vi "Sequence.vi"(8 "error in (no error)":errorcluster, 11 "Message Queues in":T62) -> (0 "error out":errorcluster)   [LabVIEW 2018, in "Sequencing Library.lvlib"]
uses:
  Sequencing Library.lvlib
  Main/Main Queue Cluster.ctl
  support/Message Queue/Message Cluster.ctl
  Drag and Drop/State Cluster.ctl
  Drag and Drop/Thumbnail Cluster.ctl
  Drag and Drop/Object Cluster.ctl
  <vilib>/Utility/miscctls.llb/LVRectTypeDef.ctl
  Drag and Drop/Object Type Enum.ctl
  <vilib>/Utility/miscctls.llb/LVPositionTypeDef.ctl
  Config Module/Controls/Main Config Cluster.ctl
  OPC/OPC Module Config.ctl
  Scale Module Folder/Measure Instrument/State Enum.ctl
  <vilib>/Utility/miscctls.llb/LVPoint32TypeDef.ctl
  OPC/OPC Settings.ctl
  OPC/Variable Data Cluster.ctl
  <vilib>/OPCUA/controls/NodeId.ctl
  <vilib>/OPCUA/controls/OPC UA StatusCode.ctl
  <vilib>/OPCUA/controls/Subscription ID.ctl
  <vilib>/OPCUA/controls/OPC UA Client Refnum.ctl
  <vilib>/OPCUA/controls/Subscription Data Change.ctl
  <vilib>/OPCUA/controls/Data Type.ctl
  Feed Module/Controls/Feed Module Config Cluster.ctl
  Feed Module/Controls/Feed Module Settings Cluster.ctl
  Ismatec ISM 831C/Controls/Ismatech Settings Cluster.ctl
  Masterflex 7550-30/Controls/Settings Cluster.ctl
  Mettler Toledo/Controls/Settings Cluster.ctl
  Bronkhorst M13 Flow Meter/Settings Cluster.ctl
  Measure Instrument/PID 2 Parameters Cluster.ctl
  Measure Instrument/PID Input Enum.ctl
  Measure Instrument/PID 2 Output Enum.ctl
  Tacmina QI/Tacmina QI DAQ Setting.ctl
  KNF Pump/Settings Cluster plus SIMDOS.ctl
  ASIA Pump/Pump Settings.ctl
  VICI M50 Party Mode/Settings Cluster.ctl
  FLOM Pump/Settings Cluster.ctl
  SSI PR Class/SSI PR Settings Cluster.ctl
  TT Module/Controls/TT Module Config Cluster.ctl
  Acquisition/Hardware Configuration.ctl
  Acquisition/Task Cluster.ctl
  PT Module/Controls/PT Module Config Cluster.ctl
  Scale Module Folder/Feed Module/Controls/Scale Module Config Cluster.ctl
  Scale Module Folder/Feed Module/Controls/Scale Module Settings Cluster.ctl
  Pump Module Folder/Pump Module Config Cluster.ctl
  Pump Module Folder/Pump Module Settings Cluster.ctl
  LabJack Module/Controls/U3 Module Config Cluster.ctl
  Decoration Module/Decoration Module Config Cluster.ctl
  Flow Module Folder/Feed Module/Controls/Flow Module Config Cluster.ctl
  Flow Module Folder/Feed Module/Controls/Flow Module Settings Cluster.ctl
  TCU Module/TCU Module Folder/TCU Module Config Cluster.ctl
  TCU Module/TCU Module Folder/TCU Module Settings Cluster.ctl
  TCU Module/TCU Module Folder/Measure Instrument/Output Devices.ctl
  Huber TCU/Huber Settings.ctl
  Lauda Integral XT-150 TCU/Lauda Settings.ctl
  Julabo Type 1 TCU/Julabo Type 1 TCU Folder/Julabo FP-50 Settings.ctl
  Huber Unistat 410 TCU/Huber Unistat 410 Settings.ctl
  D-O Module Folder/Not Sure Where this is Used.ctl
  Squence Control.ctl
  D-O Module Folder/D-O Module Config Cluster.ctl
  D-O Module Folder/Valve Clusters.ctl
  D-O Module Folder/D-O Module Settings Cluster.ctl
  D-O Module Folder/D-O Device Settings Cluster.ctl
  VICI Electronic Actuator/VICI Electronic Actuator Settings.ctl
  Pressure Regulator Control Module/Pressure Regulator/Controls/4-20mA Module Config Cluster.ctl
  Pressure Regulator Control Module/Pressure Regulator/Controls/4-20mA Module Settings Cluster.ctl
  Pressure Transmitter/Pressure Transmitter Device Settings.ctl
  Pressure Reg Module/Pressure Regulator Device Settings.ctl
  Squence Update Cluster.ctl
  support/Message Queue/Enqueue Message (Single).vi
  support/Message Queue/Message Queue.lvlib
  support/Command Log VIs/Command Logging.lvlib
  Drag and Drop/Drag and Drop.lvlib
  Config Module/Config Module.lvlib
  TT Module/TT Module.lvlib
  Feed Module/Feed Module.lvlib
  Ismatec ISM 831C/Ismatec ISM 831C.lvlib
  Masterflex 7550-30/Masterflex 7550-30.lvlib
  Mettler Toledo/Mettler Toledo.lvlib
  Bronkhorst M13 Flow Meter/Bronkhorst M13 Flow Meter.lvlib
  Tacmina QI/Tacmina QI.lvlib
  KNF Pump/KNF SIMDOS.lvlib
  ASIA Pump.lvlib
  DAQ/DAQ.lvlib
  PT Module/PT Module.lvlib
  Scale Module Folder/Scale Module.lvlib
  Pump Module Folder/Pump Module.lvlib
  LabJack Module/U3 Module.lvlib
  Flow Module Folder/Flow Module.lvlib
  TCU Module/TCU Module Folder/TCU Module.lvlib
  Huber TCU/Huber Ministat 230 TCU.lvlib
  Lauda Integral XT-150 TCU/Lauda TCU.lvlib
  Julabo Type 1 TCU/Julabo Type 1 TCU Folder/Julabo Type FP-50 TCU.lvlib
  VICI M50 Party Mode/VICI M6 M50 Party Mode.lvlib
  D-O Module Folder/D-O Module.lvlib
  Pressure Transmitter/Pressure Transmitter Library.lvlib
  Pressure Regulator Control Module/Pressure Regulator/4-20mA Module.lvlib
  Pressure Reg Module/Pressure Regulator Library.lvlib
  FLOM Pump/FLOM Pump.lvlib
  SSI PR Class/SSI PR Pump.lvlib
  Huber Unistat 410 TCU/Huber Unistat 410 TCU.lvlib
  OPC/OPC UA.lvlib
  Scale Module Folder/Measure Instrument/Scale Module Engine.lvlib
  D-O Module Folder/DIO Valve/VICI Electronic Actuator.lvlib
panel:
  out "Process Name":string
  out "Queue Name":string
  out "Loop Variable":u32
  out "Step":i32
  out "Done":bool
  out "Output":T1 {"Main Config"."PR Module Configs"."Settings"."PID 2 Parameters"."output range"."output low" format="%.2f"; "Main Config"."PR Module Configs"."Settings"."PID 2 Parameters"."output range"."output high" min=0.0 max=100.0 format="%.2f"; "Main Config"."PR Module Configs"."Settings"."PID 2 Parameters"."PID gains"."derivative time (Td, min)" format="%.3f"; "Main Config"."PR Module Configs"."Settings"."PID 2 Parameters"."PID gains"."integral time (Ti, min)" format="%.3f"; "Main Config"."PR Module Configs"."Settings"."PID 2 Parameters"."PID gains"."proportional gain (Kc)" format="%.3f"; "Main Config"."Steps"."Control" items=["Pump %", "Setpoint"]; "Main Config"."TCU Module Configs"."Settings"."Julabo FP-50 Settings"."Pump Power" min=0 max=8 step=1; "Main Config"."TCU Module Configs"."Settings"."Lauda Settings"."Pump Power" min=0 max=8 step=1; "Main Config"."Pump Module Configs"."Settings"."ASIA Pump C"."channel" min=0 max=1 step=1; "Main Config"."Pump Module Configs"."Settings"."Masterflex"."Pump Number" min=1.0 max=20.0 step=1.0; "Main Config"."Pump Module Configs"."Settings"."Ismatech"."Pump Number" min=1.0 max=20.0 step=1.0; "Main Config"."Feed Module Configs"."Settings"."output range"."output low" min=0.0 max=100.0 format="%.2f"; "Main Config"."Feed Module Configs"."Settings"."output range"."output high" format="%.2f"; "Main Config"."Feed Module Configs"."Settings"."PID 2 Parameters"."PID gains"."derivative time (Td, min)" format="%.3f"; "Main Config"."Feed Module Configs"."Settings"."PID 2 Parameters"."PID gains"."integral time (Ti, min)" format="%.3f"; "Main Config"."Feed Module Configs"."Settings"."PID 2 Parameters"."PID gains"."proportional gain (Kc)" format="%.3f"; "Main Config"."Feed Module Configs"."Settings"."ASIA Pump C"."channel" min=0 max=1 step=1; "Main Config"."Feed Module Configs"."Settings"."Ismatech"."Pump Number" min=1.0 max=20.0 step=1.0; "Main Config"."Feed Module Configs"."Settings"."Masterflex"."Pump Number" min=1.0 max=20.0 step=1.0}
  out "Intruction Cluster":T52 {"Control" items=["Setpoint", "Pump %"]}
  out "Paused":bool
  out "Stop":bool
  in  "Input":T1 {"Main Config"."PR Module Configs"."Settings"."PID 2 Parameters"."output range"."output low" format="%.2f"; "Main Config"."PR Module Configs"."Settings"."PID 2 Parameters"."output range"."output high" min=0.0 max=100.0 format="%.2f"; "Main Config"."PR Module Configs"."Settings"."PID 2 Parameters"."PID gains"."derivative time (Td, min)" format="%.3f"; "Main Config"."PR Module Configs"."Settings"."PID 2 Parameters"."PID gains"."integral time (Ti, min)" format="%.3f"; "Main Config"."PR Module Configs"."Settings"."PID 2 Parameters"."PID gains"."proportional gain (Kc)" format="%.3f"; "Main Config"."Steps"."Control" items=["Pump %", "Setpoint"]; "Main Config"."TCU Module Configs"."Settings"."Julabo FP-50 Settings"."Pump Power" min=0 max=8 step=1; "Main Config"."TCU Module Configs"."Settings"."Lauda Settings"."Pump Power" min=0 max=8 step=1; "Main Config"."Pump Module Configs"."Settings"."ASIA Pump C"."channel" min=0 max=1 step=1; "Main Config"."Pump Module Configs"."Settings"."Masterflex"."Pump Number" min=1.0 max=20.0 step=1.0; "Main Config"."Pump Module Configs"."Settings"."Ismatech"."Pump Number" min=1.0 max=20.0 step=1.0; "Main Config"."Feed Module Configs"."Settings"."output range"."output low" min=0.0 max=100.0 format="%.2f"; "Main Config"."Feed Module Configs"."Settings"."output range"."output high" format="%.2f"; "Main Config"."Feed Module Configs"."Settings"."PID 2 Parameters"."PID gains"."derivative time (Td, min)" format="%.3f"; "Main Config"."Feed Module Configs"."Settings"."PID 2 Parameters"."PID gains"."integral time (Ti, min)" format="%.3f"; "Main Config"."Feed Module Configs"."Settings"."PID 2 Parameters"."PID gains"."proportional gain (Kc)" format="%.3f"; "Main Config"."Feed Module Configs"."Settings"."ASIA Pump C"."channel" min=0 max=1 step=1; "Main Config"."Feed Module Configs"."Settings"."Ismatech"."Pump Number" min=1.0 max=20.0 step=1.0; "Main Config"."Feed Module Configs"."Settings"."Masterflex"."Pump Number" min=1.0 max=20.0 step=1.0}
  # "Instrument Settings"
  # "Instrument Settings"
  # "Output Instruments"
  # "Flow Meter Settings"
  # "Output Instruments"
  # "Scale Settings"
  # "Output Instruments"
  # "Input Instruments"
  # "Instrument Settings"
  # "Instrument Settings"
  # "Output Instruments"
  # "Flow Meter Settings"
  # "Output Instruments"
  # "Scale Settings"
  # "Output Instruments"
  # "Input Instruments"
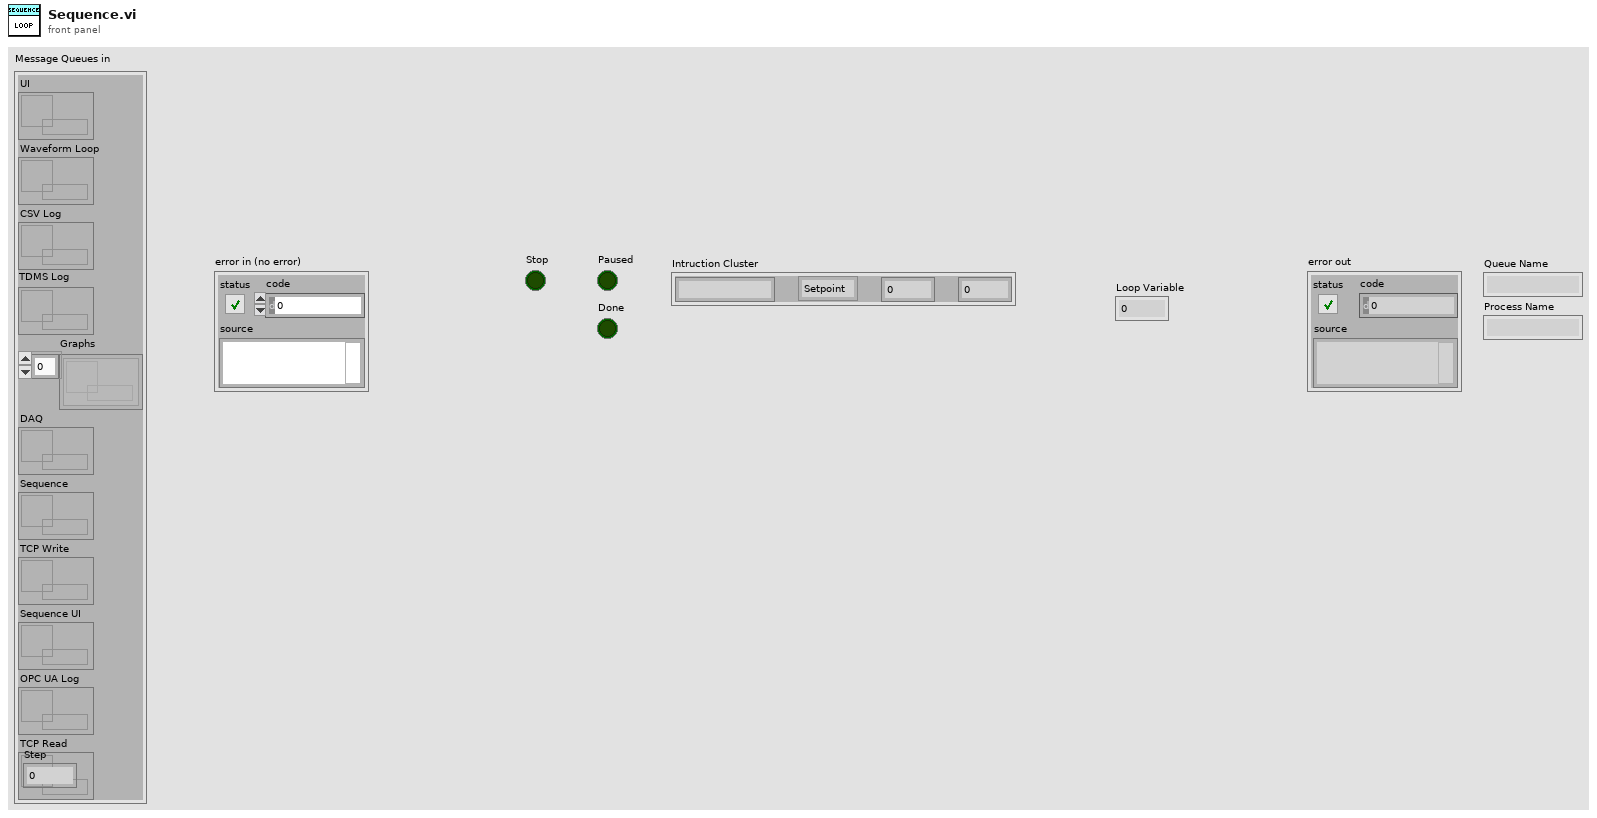
[diagram p1: front panel]
types:
  T1 = typedef "Drag and Drop.lvlib/State Cluster.ctl" = cluster{"VI refs":refnum<vi>[], "Queues":refnum<queue>[], "[Thumbnails]":T2[], "Drag Object Idx":i32, "[Objects]":T3[], "Active Object":i32, "Drop Offset":T6, "Process Name":string, "Main Config":T7, "Campaign Filepath":path, "Config Changed?":bool}
  T2 = typedef "Thumbnail Cluster.ctl" = cluster{"Path":path, "Rectangle":cluster{"left":i16, "top":i16, "right":i16, "bottom":i16}}
  T3 = typedef "Object Cluster.ctl" = cluster{"BMP Path":path, "Anchor Position":cluster{"X":i32, "Y":i32}, "Hot Spot":T4, "Type":T5, "Parameters":variant}
  T4 = typedef "LVRectTypeDef.ctl" = cluster{"Left":i16, "Top":i16, "Right":i16, "Bottom":i16}
  T5 = typedef "Object Type Enum.ctl" = enum16{"Icon", "Line", "Text", "Feed Module"}
  T6 = typedef "LVPositionTypeDef.ctl" = cluster{"Left":i32, "Top":i32}
  T7 = typedef "Config Module.lvlib/Main Config Cluster.ctl" = cluster{"OPC Module Configs":T8[], "Feed Module Configs":T17[], "Log File Path":path, "TT Module Configs":T32[], "DAQ Config":T33, "PT Module Configs":T35[], "Scale Module Configs":T36[], "Pump Module Configs":T38[], "U3 Module Configs":T40[], "Decoration Module Configs":T41[], "Flow Module Configs":T42[], "TCU Module Configs":T44[], "Steps":T51, "Abort":bool, "DO Module Configs":T53[], "PR Module Configs":T58[], "Cycle Period":dbl}
  T8 = typedef "OPC UA.lvlib/OPC Module Config.ctl" = cluster{"State":T9, "GUID":string, "Drop Coords":T10, "Configuration":T11, "First Iteration":bool, "Data":cluster{"Object Name":string, "Variable Array":T12[]}[], "Process Name":string, "Load Count":i32, "Log Started":bool, "subscription ID out":T15, "OPC UA client refnum out":T16, "Event Registration Refnum":refnum<event-registration>, "Start Time":timestamp, "Current Time":timestamp}
  T9 = typedef "Scale Module.lvlib/Scale Module Engine.lvlib/State Enum.ctl" = enum16{"Measuring", "Idle"}
  T10 = typedef "LVPoint32TypeDef.ctl" = cluster{"Horizontal":i32, "Vertical":i32}
  T11 = typedef "OPC UA.lvlib/OPC Settings.ctl" = cluster{"Cycle Period":dbl, "server endpoint URL":string, "security policy":cluster{"message mode":enum16{"None", "Sign", "Sign and Encrypt"}, "security":enum16{"Basic256", "Basic128Rsa15"}}, "Trust Any Server":bool}
  T12 = typedef "OPC UA.lvlib/Variable Data Cluster.ctl" = cluster{"node ID":T13, "browse name":string, "status":T14, "timestamp":timestamp, "value ":variant}
  T13 = typedef "NodeId.ctl" = string
  T14 = typedef "OPC UA StatusCode.ctl" = u32
  T15 = typedef "Subscription ID.ctl" = u32
  T16 = typedef "OPC UA Client Refnum.ctl" = refnum<k21>
  T17 = typedef "Feed Module.lvlib/Feed Module Config Cluster.ctl" = cluster{"GUID":string, "Drop Coords":T10, "Process Name":string, "Queue Name":string, "Settings":T18, "Settings Load Count":i32, "OP Load Count":i32}
  T18 = typedef "Feed Module.lvlib/Feed Module Settings Cluster.ctl" = cluster{"Cycle Period":dbl, "Ismatech":T19, "Masterflex":T20, "Mettler":T21, "Bronkhorst M13 Flow Meter":T22, "PID 2 Parameters":T23, "Manual Entry":dbl, "Auto?":bool, "output range":cluster{"output high":dbl, "output low":dbl}, "Bronkhorst M14":T21, "Tacmina Settings":T26, "KNF SIMDOS Settings":T27, "ASIA Pump C":T28, "VICI Settings":T29, "FLOM Settings":T30, "SSI PR Settings":T31}
  T19 = typedef "Ismatec ISM 831C.lvlib/Ismatech Settings Cluster.ctl" = cluster{"VISA resource name":refnum<visa-resource-name>, "Simulated?":bool, "Pump Number":dbl, "Reverse?":bool}
  T20 = typedef "Masterflex 7550-30.lvlib/Settings Cluster.ctl" = cluster{"VISA resource name":refnum<visa-resource-name>, "Simulated?":bool, "Pump Number":dbl, "Reverse?":bool}
  T21 = typedef "Mettler Toledo.lvlib/Settings Cluster.ctl" = cluster{"VISA resource name":refnum<visa-resource-name>, "Simulated?":bool}
  T22 = typedef "Bronkhorst M13 Flow Meter.lvlib/Settings Cluster.ctl" = cluster{"VISA resource name":refnum<visa-resource-name>, "Simulated?":bool}
  T23 = typedef "PID 2 Parameters Cluster.ctl" = cluster{"Input Device":T24, "Output Device":T25, "Setpoint":dbl, "PID gains":cluster{"proportional gain (Kc)":dbl, "integral time (Ti, min)":dbl, "derivative time (Td, min)":dbl}}
  T24 = typedef "PID Input Enum.ctl" = enum16{"Default", "Bronkhorst M13", "Bronkhorst M14", "Scale Rate of Change"}
  T25 = typedef "PID 2 Output Enum.ctl" = enum16{"Default", "Ismatec ISM 831C", "Masterflex 7550-30", "VICI", "Tacmina QI", "KNF SIMDOS", "ASIA Type C", "FLOM UI-22-11", "SSI PR"}
  T26 = typedef "Tacmina QI.lvlib/Tacmina QI DAQ Setting.ctl" = cluster{"Analog DAQ Task":refnum<k21>, "Digital DAQ Task":refnum<k21>}
  T27 = typedef "KNF SIMDOS.lvlib/Settings Cluster plus SIMDOS.ctl" = cluster{"VISA resource name":refnum<visa-resource-name>, "Simulated?":bool}
  T28 = typedef "ASIA Pump.lvlib/Pump Settings.ctl" = cluster{"ASIA Pump #":i32, "channel":i32, "Simulated":bool}
  T29 = typedef "VICI M6 M50 Party Mode.lvlib/Settings Cluster.ctl" = cluster{"VISA resource name":refnum<visa-resource-name>, "Simulated?":bool, "Pump Letter":string, "Reverse?":bool}
  T30 = typedef "FLOM Pump.lvlib/Settings Cluster.ctl" = cluster{"VISA resource name":refnum<visa-resource-name>, "Simulated?":bool, "Pump Number":dbl}
  T31 = typedef "SSI PR Pump.lvlib/SSI PR Settings Cluster.ctl" = cluster{"VISA resource name":refnum<visa-resource-name>, "Simulated?":bool}
  T32 = typedef "TT Module.lvlib/TT Module Config Cluster.ctl" = cluster{"GUID":string, "Drop Coords":T10, "Input Channel Tag Name ":string, "Process Name":string, "Queue Name":string, "Input Channel Numeric Alarm Settings":cluster{"enable? (F)":bool, "name":string, "alarm type":enum16{"HI_HI", "HI", "LO", "LO_LO"}, "level/change":dbl, "deadband/time":dbl, "priority":u32, "ack type":enum16{"Auto", "User", "None", "Each Occurrence"}, "area":string, "description":string, "log? (T)":bool}[]}
  T33 = typedef "DAQ.lvlib/Hardware Configuration.ctl" = cluster{"Tasks":T34[]}
  T34 = typedef "Task Cluster.ctl" = cluster{"DAQmx Task":refnum<k21>, "Read-Write Radio":enum32{"Read", "Write"}}
  T35 = typedef "PT Module.lvlib/PT Module Config Cluster.ctl" = cluster{"GUID":string, "Drop Coords":T10, "Input Channel Tag Name ":string, "Process Name":string, "Queue Name":string, "Input Channel Numeric Alarm Settings":cluster{"enable? (F)":bool, "name":string, "alarm type":enum16{"HI_HI", "HI", "LO", "LO_LO"}, "level/change":dbl, "deadband/time":dbl, "priority":u32, "ack type":enum16{"Auto", "User", "None", "Each Occurrence"}, "area":string, "description":string, "log? (T)":bool}[]}
  T36 = typedef "Scale Module.lvlib/Scale Module Config Cluster.ctl" = cluster{"GUID":string, "Drop Coords":T10, "Process Name":string, "Queue Name":string, "Settings":T37, "Load Count":i32}
  T37 = typedef "Scale Module.lvlib/Scale Module Settings Cluster.ctl" = cluster{"Cycle Period":dbl, "Mettler":T21, "Scale Type":string}
  T38 = typedef "Pump Module.lvlib/Pump Module Config Cluster.ctl" = cluster{"GUID":string, "Drop Coords":T10, "Process Name":string, "Queue Name":string, "Settings":T39, "Load Count":i32}
  T39 = typedef "Pump Module.lvlib/Pump Module Settings Cluster.ctl" = cluster{"Cycle Period":dbl, "Ismatech":T19, "Masterflex":T20, "Manual Entry":dbl, "VICI Settings":T29, "Output Device":T25, "Tacmina Settings":T26, "KNF SIMDOS Settings":T27, "ASIA Pump C":T28, "FLOM Settings":T30, "Pump Calibration File":path, "Calibration":dbl, "Pump Cal Enum":u16, "SSI PR Settings":T31}
  T40 = typedef "U3 Module.lvlib/U3 Module Config Cluster.ctl" = cluster{"GUID":string, "Drop Coords":T10, "AI Channel Number":enum16{"Default", "AI0", "AI1", "AI2", "AI3", "AI4", "AI5", "AI6", "AI7"}, "Process Name":string, "Queue Name":string, "Input Channel Numeric Alarm Settings":cluster{"enable? (F)":bool, "name":string, "alarm type":enum16{"HI_HI", "HI", "LO", "LO_LO"}, "level/change":dbl, "deadband/time":dbl, "priority":u32, "ack type":enum16{"Auto", "User", "None", "Each Occurrence"}, "area":string, "description":string, "log? (T)":bool}[]}
  T41 = typedef "Decoration Module Config Cluster.ctl" = cluster{"GUID":string, "Drop Coords":T10, "Decoration Filepath":path}
  T42 = typedef "Flow Module.lvlib/Flow Module Config Cluster.ctl" = cluster{"GUID":string, "Drop Coords":T10, "Process Name":string, "Queue Name":string, "Settings":T43, "Load Count":i32}
  T43 = typedef "Flow Module.lvlib/Flow Module Settings Cluster.ctl" = cluster{"Cycle Period":dbl, "Bronkhorst M13":T21, "Flow Meter Type":string, "Bronkhorst M14":T21}
  T44 = typedef "TCU Module.lvlib/TCU Module Config Cluster.ctl" = cluster{"GUID":string, "Drop Coords":T10, "Process Name":string, "Queue Name":string, "Settings":T45, "Load Count":i32, "Power Level Changed":bool}
  T45 = typedef "TCU Module.lvlib/TCU Module Settings Cluster.ctl" = cluster{"Cycle Period":dbl, "Setpoint Entry":dbl, "Output Device":T46, "Huber Ministat 230 Settings":T47, "Lauda Settings":T48, "Julabo FP-50 Settings":T49, "Internal Control?":bool, "Huber Unistat 410 Settings":T50}
  T46 = typedef "Output Devices.ctl" = enum16{"Default", "Huber Ministat 230", "Huber Unistat 410", "Lauda XT-150", "Julabo FP-50"}
  T47 = typedef "Huber Ministat 230 TCU.lvlib/Huber Settings.ctl" = cluster{"VISA resource name":refnum<visa-resource-name>, "Simulated?":bool}
  T48 = typedef "Lauda TCU.lvlib/Lauda Settings.ctl" = cluster{"VISA resource name":refnum<visa-resource-name>, "Simulated?":bool, "Pump Power":i32}
  T49 = typedef "Julabo Type FP-50 TCU.lvlib/Julabo FP-50 Settings.ctl" = cluster{"VISA resource name":refnum<visa-resource-name>, "Simulated?":bool, "Pump Power":i32}
  T50 = typedef "Huber Unistat 410 TCU.lvlib/Huber Unistat 410 Settings.ctl" = cluster{"VISA resource name":refnum<visa-resource-name>, "Simulated?":bool}
  T51 = typedef "Not Sure Where this is Used.ctl" = T52[]
  T52 = typedef "Sequencing Library.lvlib/Squence Control.ctl" = cluster{"Module":string, "Control":u16, "Value":dbl, "Wait (sec)":dbl}
  T53 = typedef "D-O Module.lvlib/D-O Module Config Cluster.ctl" = cluster{"GUID":string, "Drop Coords":T10, "Process Name":string, "Queue Name":string, "Settings":T54, "Load Count":i32}
  T54 = typedef "D-O Module.lvlib/Valve Clusters.ctl" = cluster{"Valve Settings":T55, "Valve Type":enum16{"Default", "Digital Output Valve", "VICI Electronic Actuator"}, "Time On (Sec)":dbl, "Time Off (Sec)":dbl, "Run?":bool}
  T55 = typedef "D-O Module.lvlib/D-O Module Settings Cluster.ctl" = cluster{"D-O Settings":T56, "VICI Electronic Actuator":T57}
  T56 = typedef "D-O Module.lvlib/D-O Device Settings Cluster.ctl" = cluster{"DAQmx Task Name":refnum<k21>, "Output Channel":u16, "Output Channel Names":string[]}
  T57 = typedef "VICI Electronic Actuator.lvlib/VICI Electronic Actuator Settings.ctl" = cluster{"VISA resource name":refnum<visa-resource-name>, "Mode":enum16{"Two Positions With Stops", "Two Positions Without Stops", "Mutiposition"}, "Simulated":bool}
  T58 = typedef "4-20mA Module.lvlib/4-20mA Module Config Cluster.ctl" = cluster{"GUID":string, "Drop Coords":T10, "Process Name":string, "Queue Name":string, "Settings":T59, "Settings Load Count":i32}
  T59 = typedef "4-20mA Module.lvlib/4-20mA Module Settings Cluster.ctl" = cluster{"Cycle Period":dbl, "PID 2 Parameters":cluster{"Input Device":enum16{"Default", "4-20mA"}, "Output Device":enum16{"Default", "Equilibar Pressure Reg", "Flow Regulator"}, "Setpoint":dbl, "PID gains":cluster{"proportional gain (Kc)":dbl, "integral time (Ti, min)":dbl, "derivative time (Td, min)":dbl}, "output range":cluster{"output low":dbl, "output high":dbl}}, "Manual Entry":dbl, "Auto?":bool, "4-20mA Input Settings":T60, "4-20mA Out Settings":T61, "Input Channel Tag Name ":string}
  T60 = typedef "Pressure Transmitter Library.lvlib/Pressure Transmitter Device Settings.ctl" = cluster{"Input Channel ":u16}
  T61 = typedef "Pressure Regulator Library.lvlib/Pressure Regulator Device Settings.ctl" = cluster{"Output DAQ Task":refnum<k21>}
  T62 = typedef "Main Queue Cluster.ctl" = cluster{"UI":refnum<queue>, "Waveform Loop":refnum<queue>, "CSV Log":refnum<queue>, "TDMS Log":refnum<queue>, "Graphs":refnum<queue>[], "DAQ":refnum<queue>, "Sequence":refnum<queue>, "TCP Write":refnum<queue>, "Sequence UI":refnum<queue>, "OPC UA Log":refnum<queue>, "TCP Read":refnum<queue>}
  T63 = typedef "Sequencing Library.lvlib/Squence Update Cluster.ctl" = cluster{"Auto?":bool, "Manual Entry":dbl, "Setpoint":dbl}
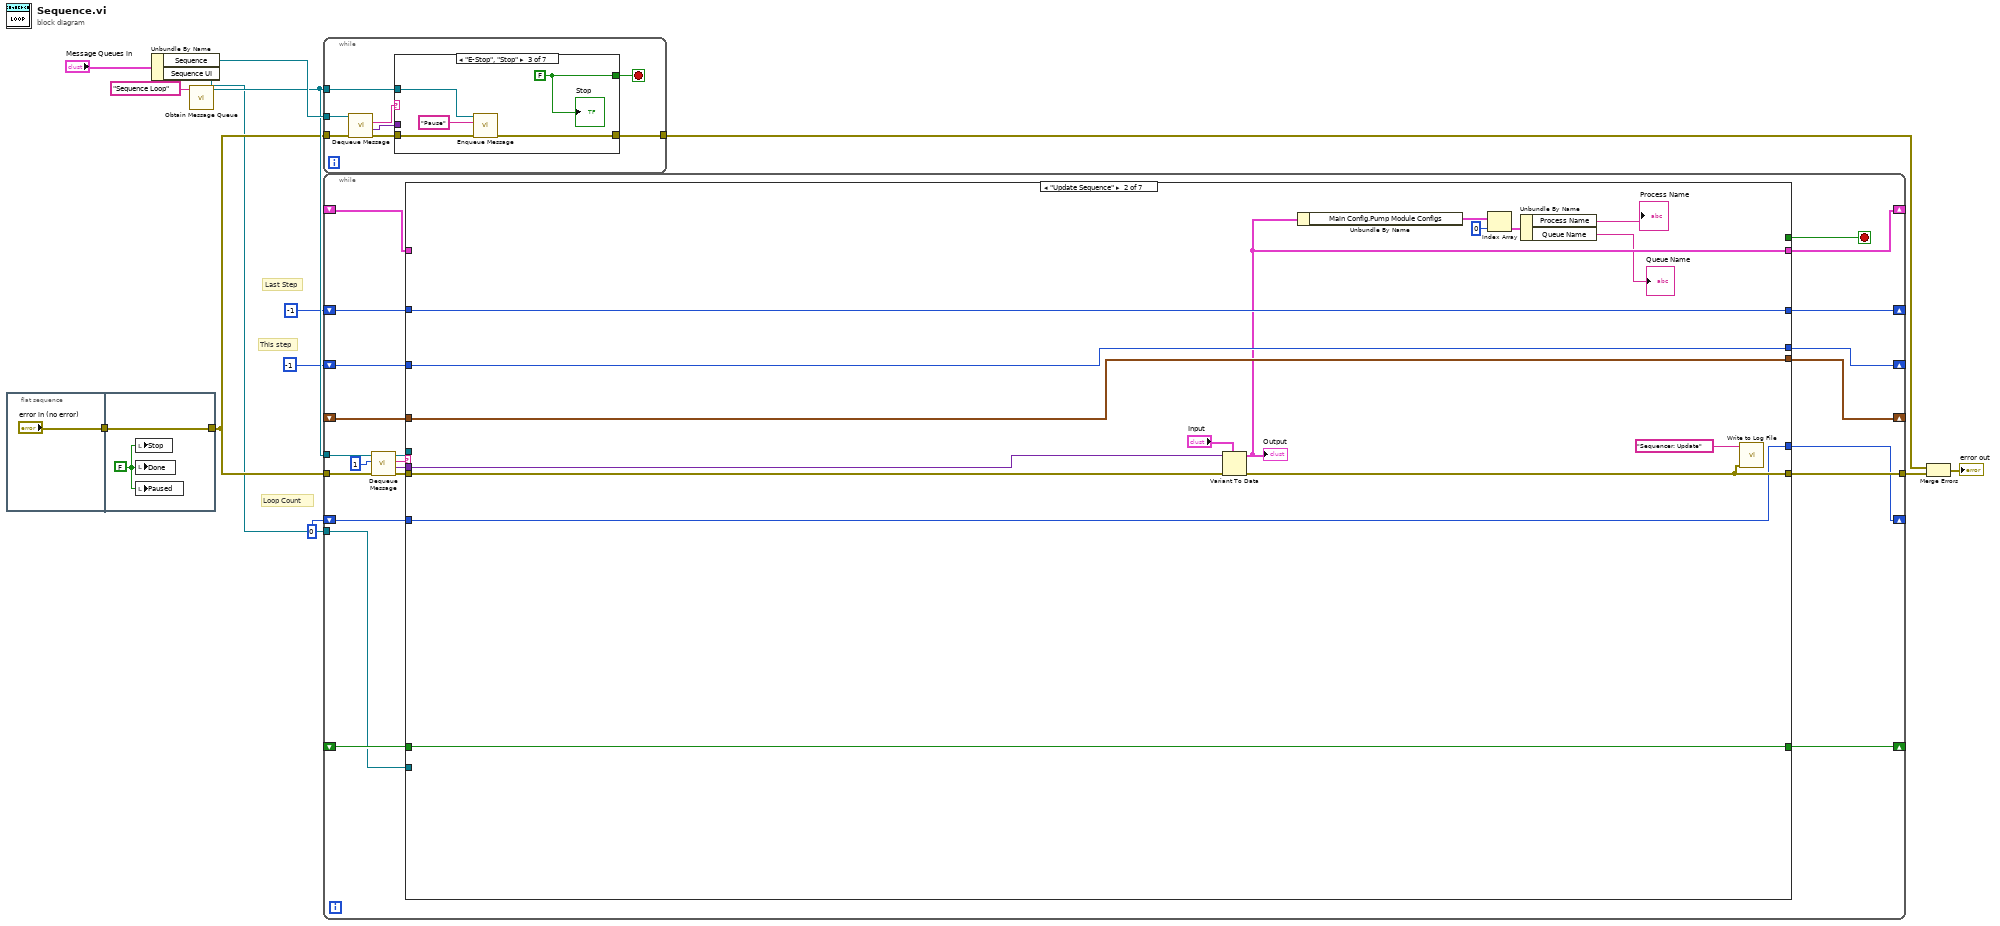
[diagram p0: block diagram]
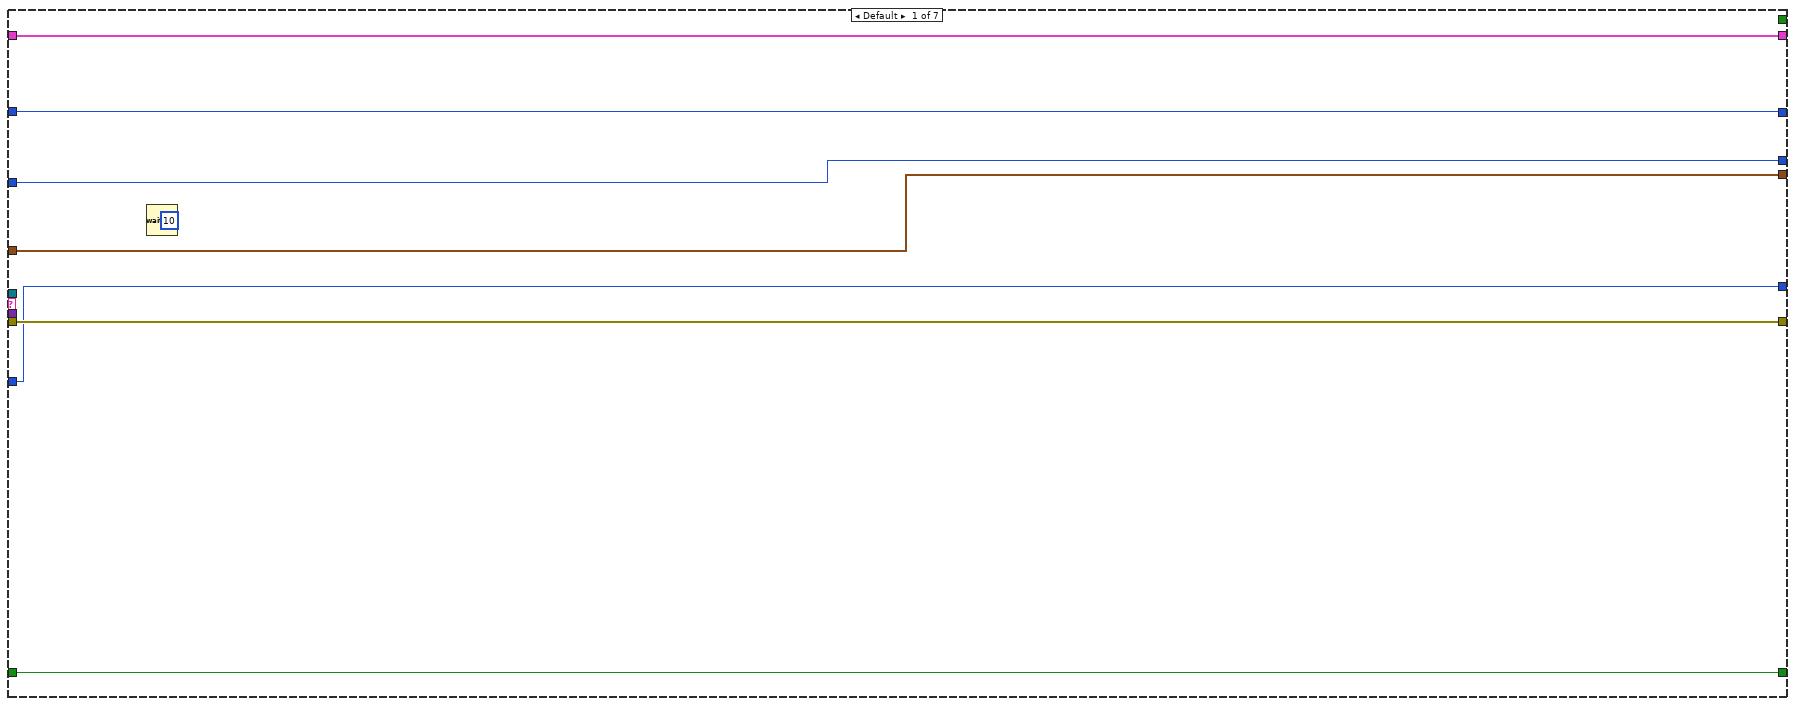
[diagram p2: hidden frame]
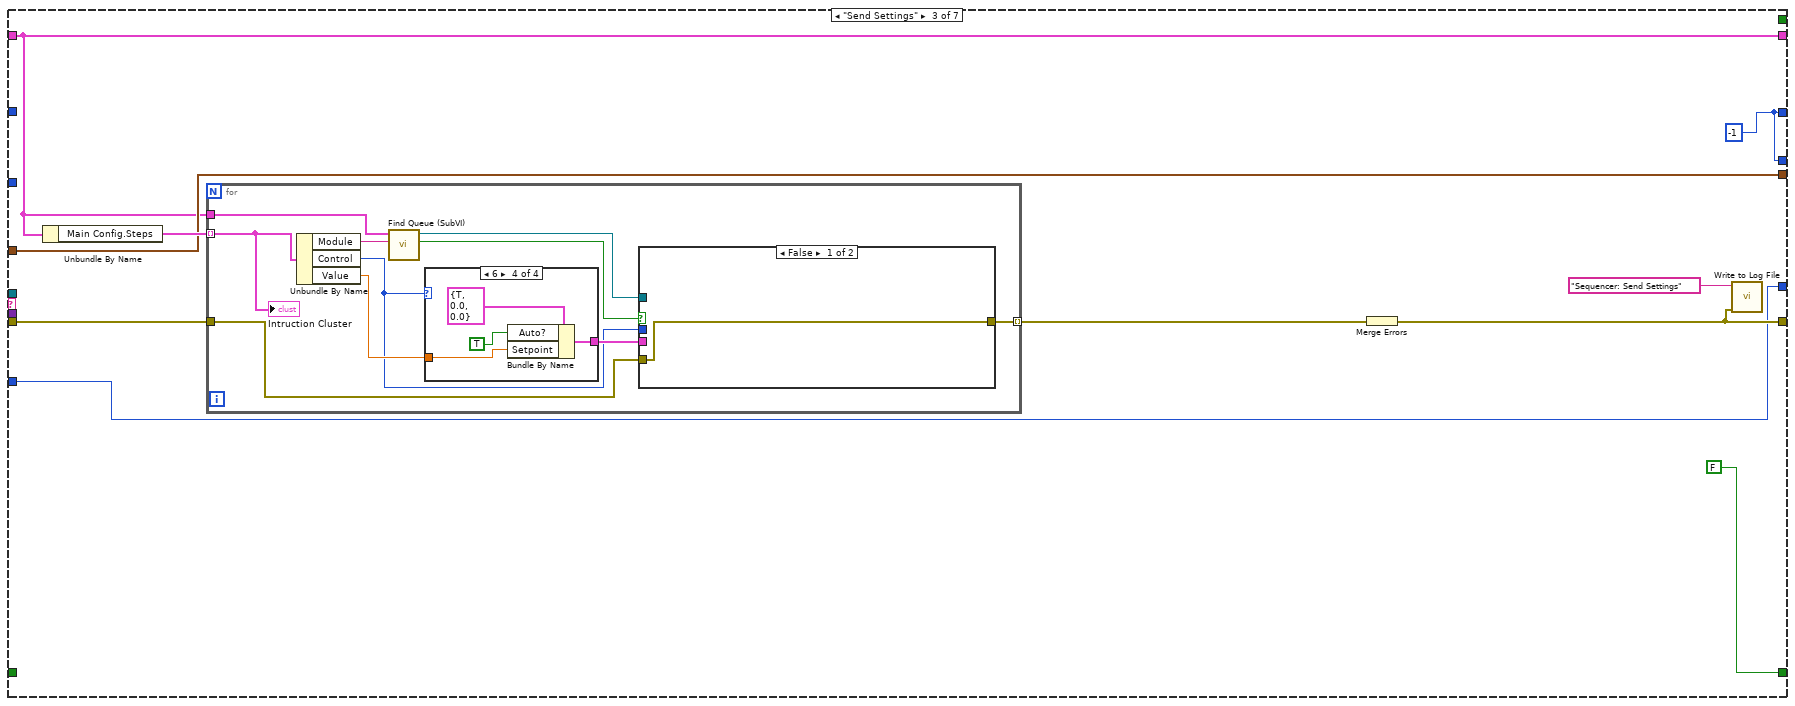
[diagram p3: hidden frame]
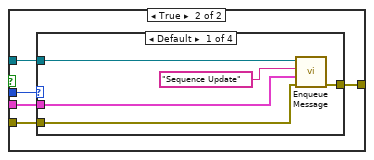
[diagram p4: hidden frame]
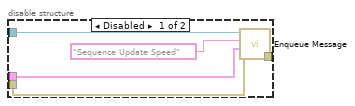
[diagram p7: hidden frame]
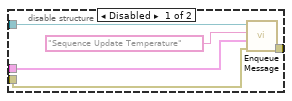
[diagram p9: hidden frame]
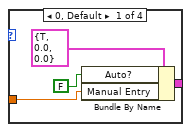
[diagram p10: hidden frame]
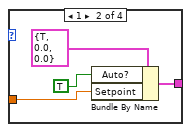
[diagram p11: hidden frame]
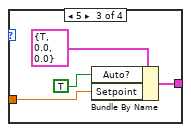
[diagram p12: hidden frame]
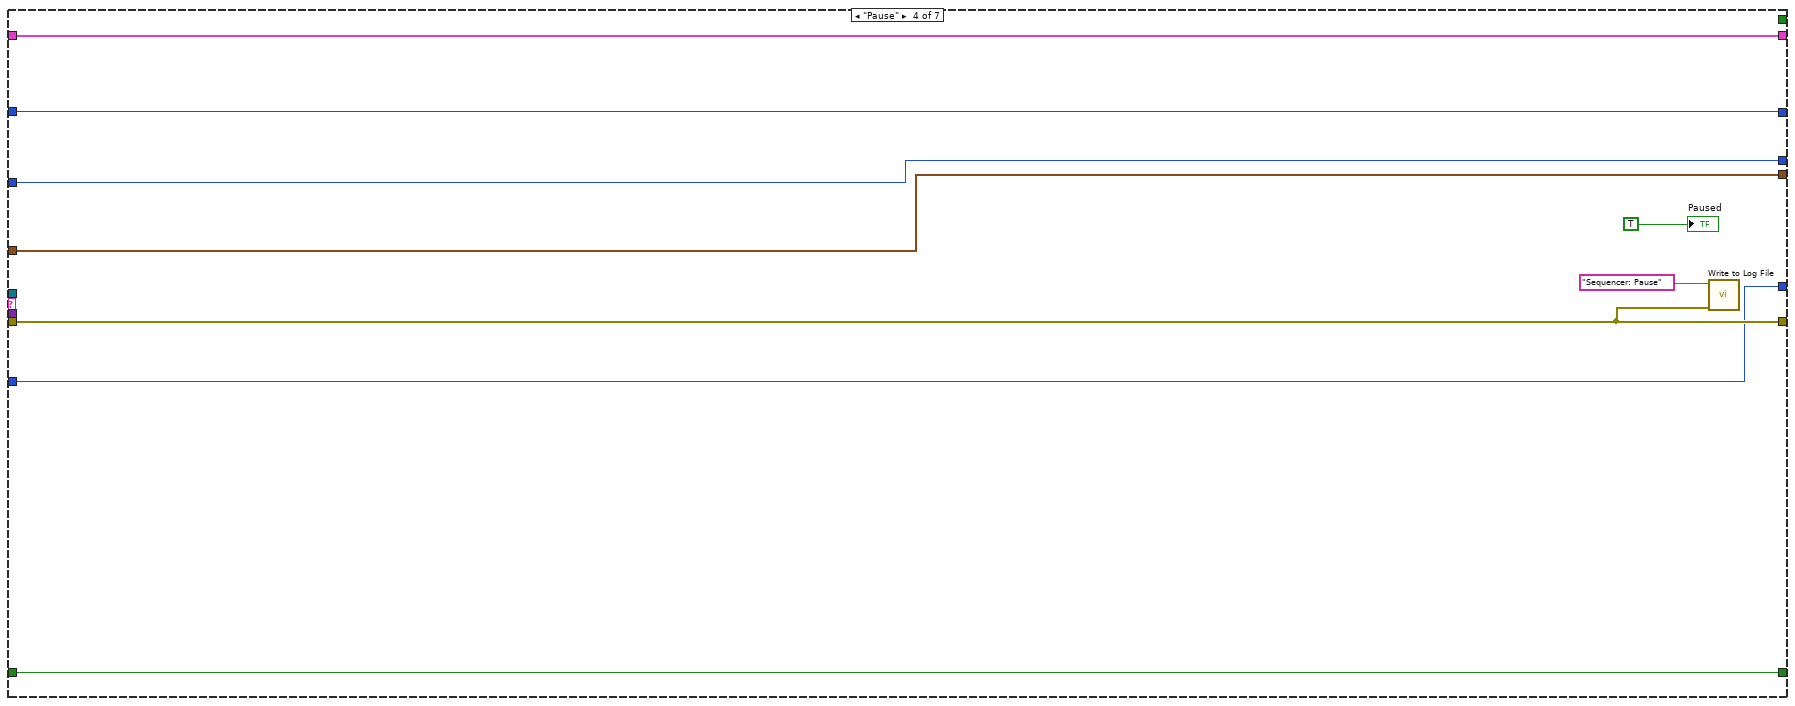
[diagram p13: hidden frame]
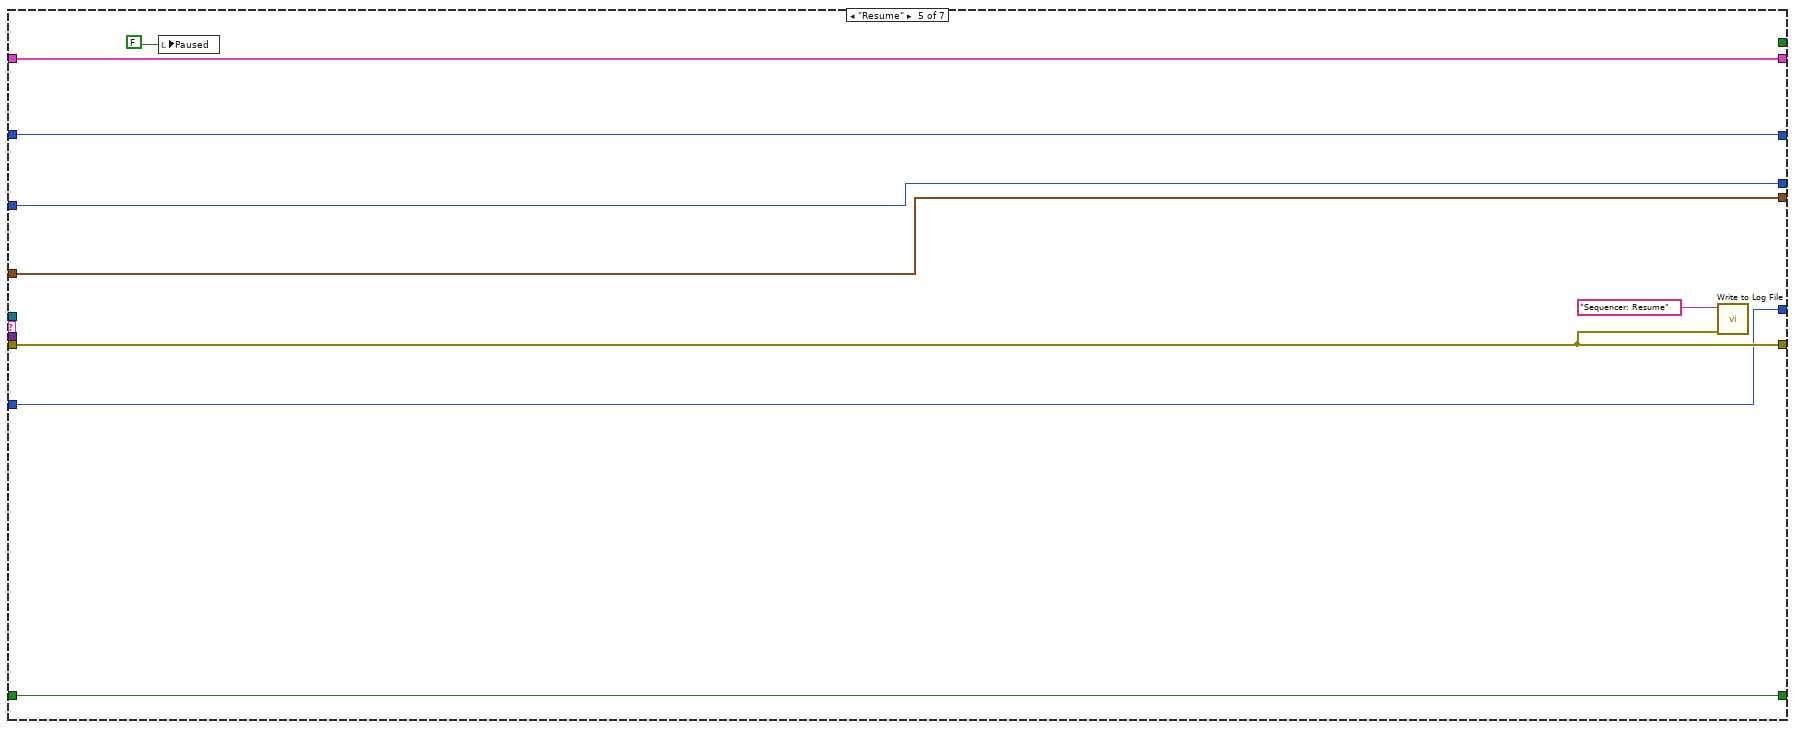
[diagram p14: hidden frame]
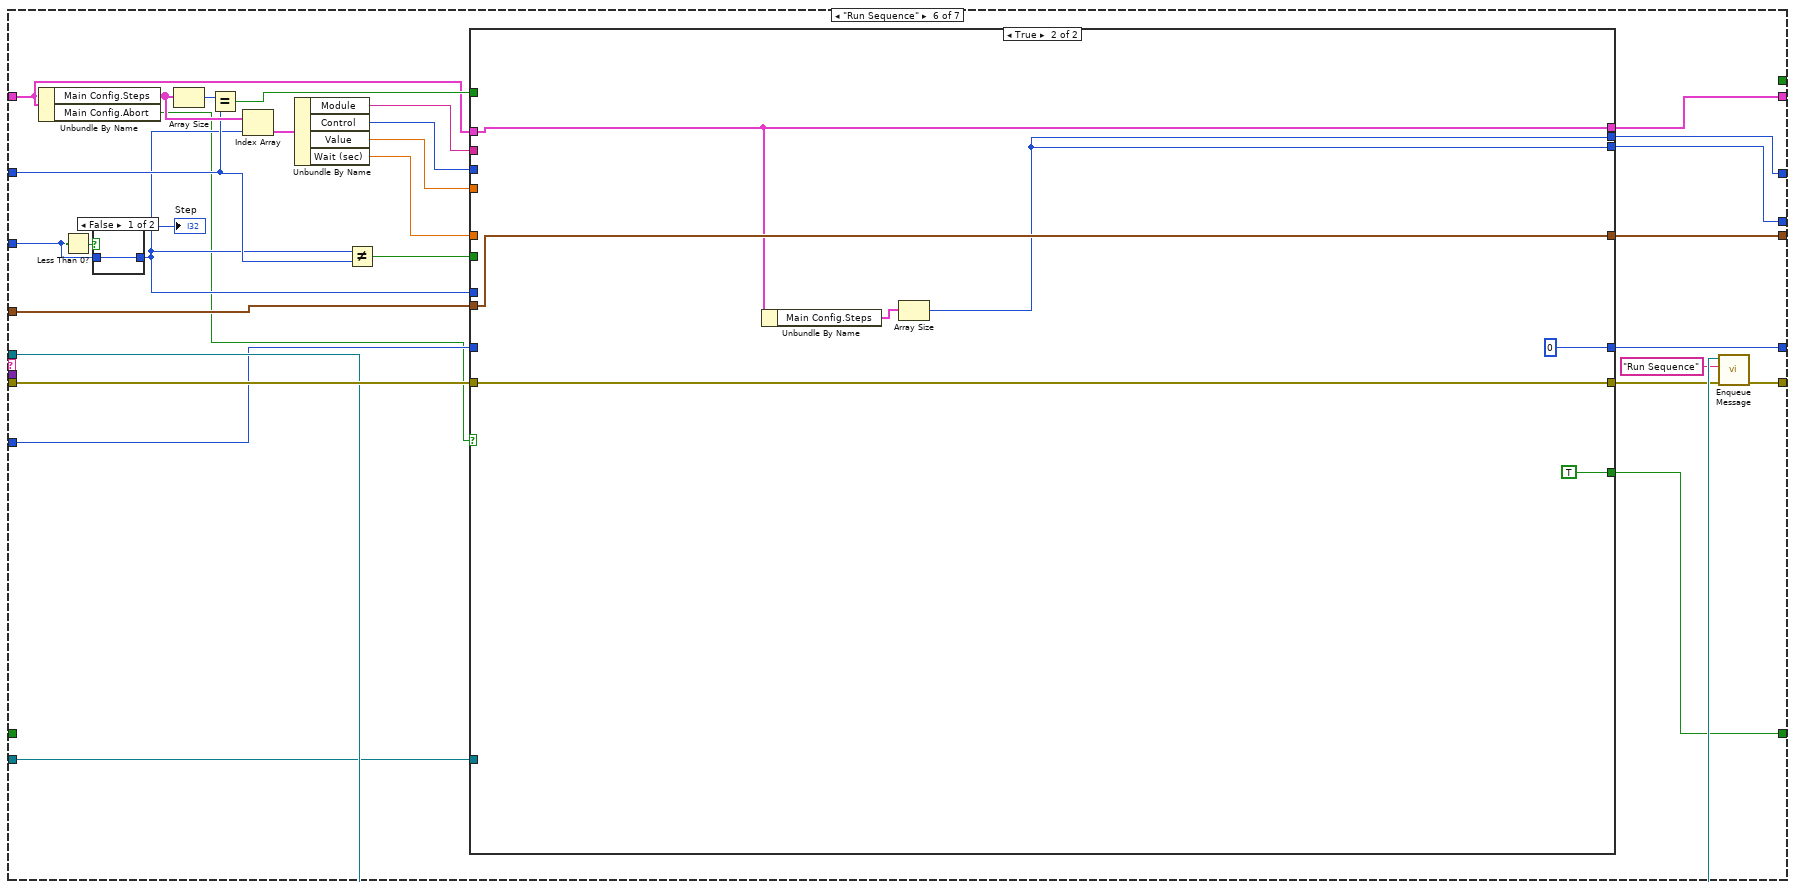
[diagram p15: hidden frame]
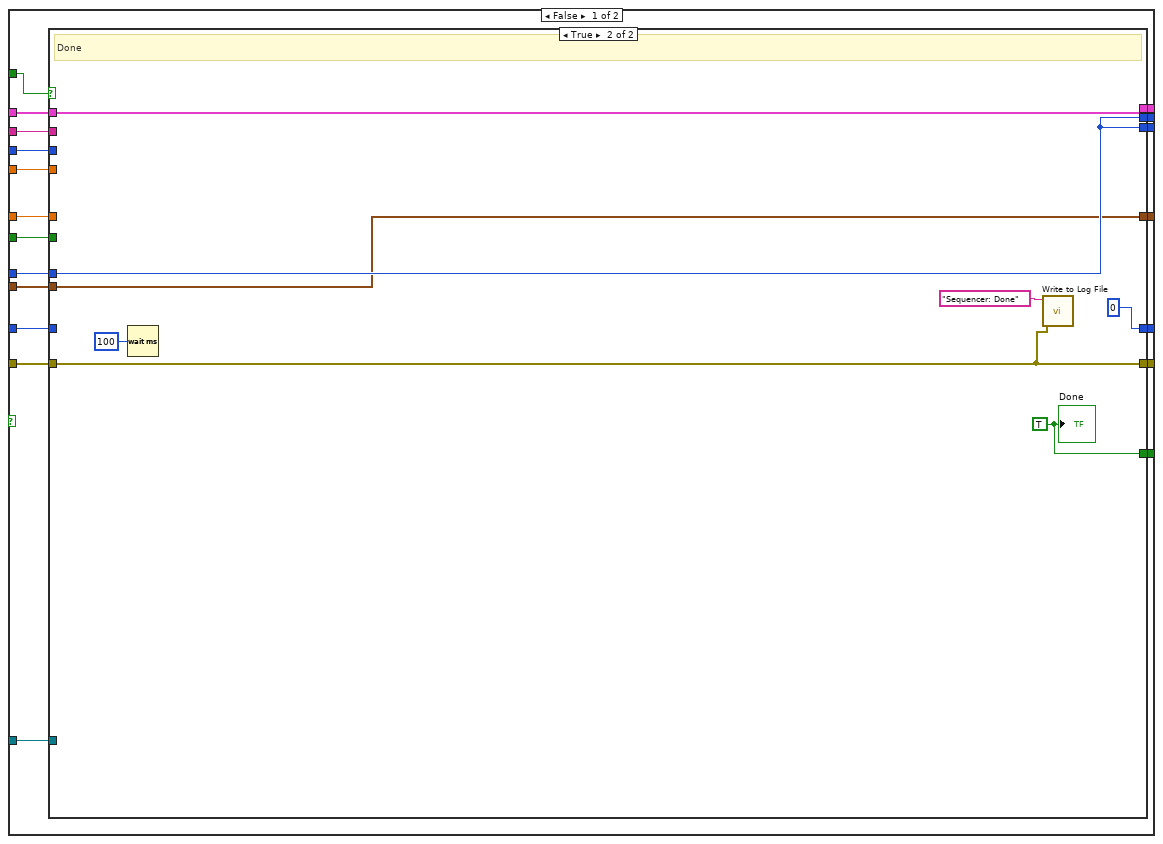
[diagram p16: hidden frame]
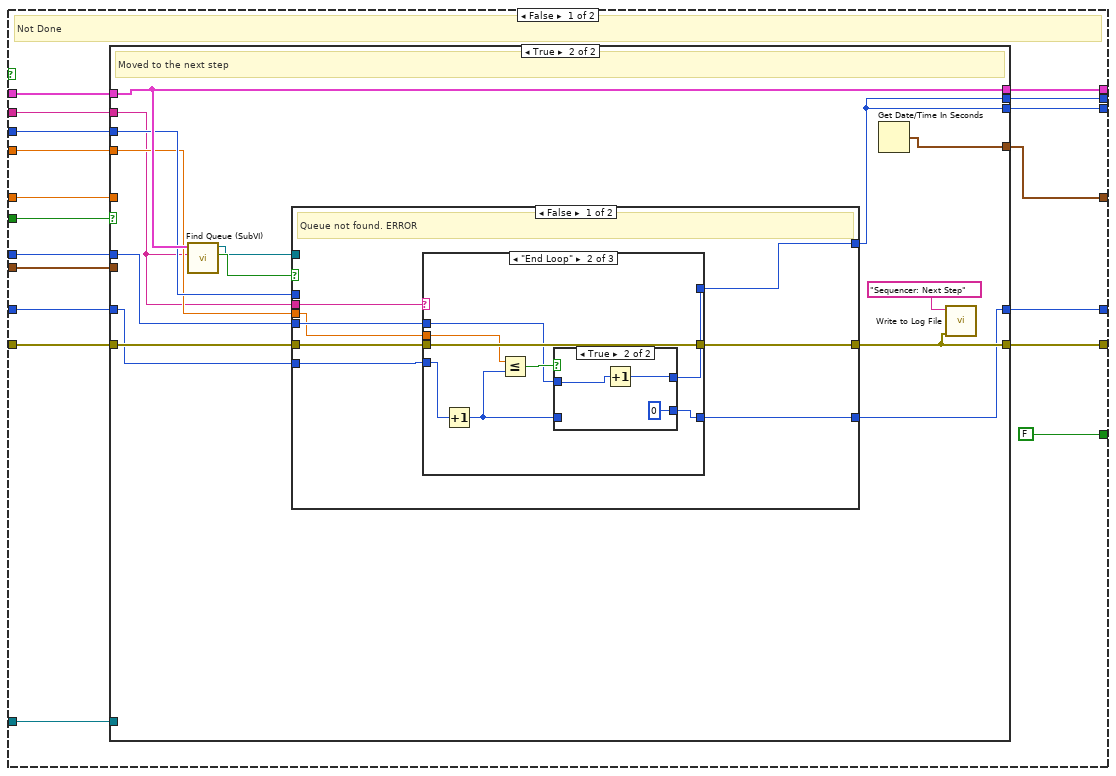
[diagram p17: hidden frame]
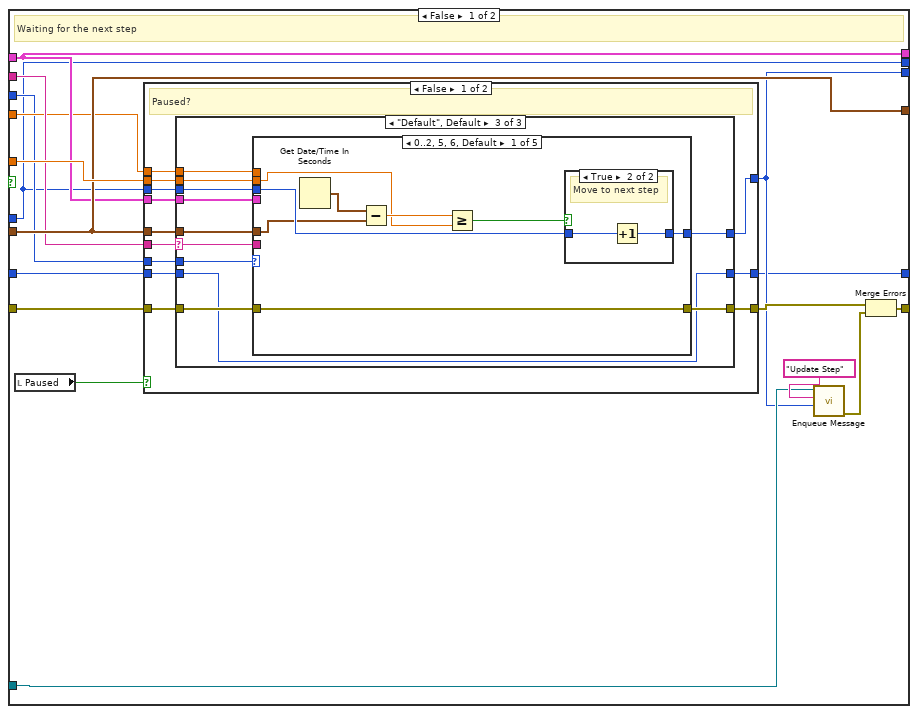
[diagram p18: hidden frame]
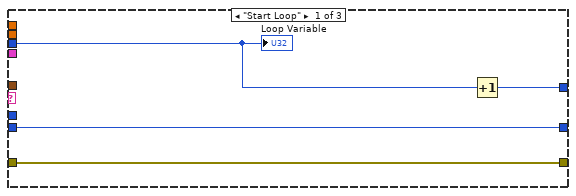
[diagram p19: hidden frame]
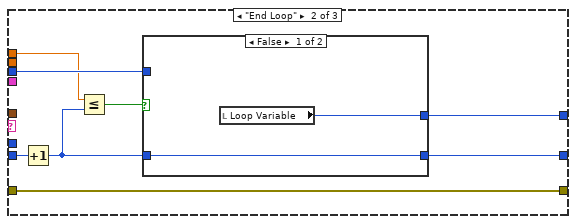
[diagram p20: hidden frame]
diagram:
  # "Loop Count"
  # "This step"
  # "Last Step"
  n1 = flat-sequence {
    tunnel: ["error in (no error)"] -> w1
    tunnel: [w16] -> w9
    tunnel: w1 -> [w16]
    frame #0 {
    }
    frame #1 {
      w15 = FALSE ("Paused")
      n2 = local write "Stop"(w15) -> ()
      n3 = local write "Done"(w15) -> ()
      n4 = local write "Paused"(w15) -> ()
    }
  }
  n5 = Unbundle By Name("Message Queues in") -> ("Sequence"=w12:refnum<queue>, "Sequence UI"=w3:refnum<queue>)
  n6 = call "Obtain Message Queue.vi"("name (unnamed)"="Sequence Loop") -> ("Message Queue"=w10:refnum<queue>)  [unwired: 9 in, 1 out]
  n7 = while {
    tunnel: w12 -> [w24]
    tunnel: w9 -> [w20]
    tunnel: [w21] -> w8
    tunnel: w10 -> [w17]
    stop <- w18 stop-if-true
    n8 = call "Dequeue Message.vi"("error in (no error)"=w20, "Message Queue"=w24) -> ("error out"=w19:errorcluster, "Message Data"=w22:variant, "Message"=w23:string)  [unwired: 6 in, 1 out]
    n9 = case shown="\"E-Stop\", \"Stop\"" w23 {
      tunnel: w22 -> [_ _ _ _ w43 w48 w53]
      tunnel: w19 -> [w25 w32 w36 w41 w45 w50 w55]
      tunnel: [w25 w26 w35 w40 w44 w49 w54] -> w21
      tunnel: [_ _ w33 w38 _ _ _] -> w18
      tunnel: w17 -> [_ w30 w34 w39 w46 w51 w56]
      frame Default {
      }
      frame "Start Sequence" {
        n10 = call-poly "Enqueue Message.vi"("error in (no error)"=w32, "Message"="Send Settings", "Message Queue"=w30) -> ("error out"=w27:errorcluster, "dup Message Queue"=w29:refnum<queue>)  [unwired: 7 in]
        n11 = call-poly "Enqueue Message.vi"("error in (no error)"=w27, "Message"="Run Sequence", "Message Queue"=w29) -> ("error out"=w26:errorcluster)  [unwired: 7 in, 1 out]
      }
      frame "E-Stop", "Stop" {
        w33 = FALSE
        n12 = call-poly "Enqueue Message.vi"("error in (no error)"=w36, "Message"="Pause", "Message Queue"=w34) -> ("error out"=w35:errorcluster)  [unwired: 7 in, 1 out]
        "Stop" <- w33
      }
      frame "Exit" {
        w38 = TRUE
        n13 = call-poly "Enqueue Message.vi"("error in (no error)"=w41, "Message"="Exit", "Message Queue"=w39) -> ("error out"=w40:errorcluster)  [unwired: 7 in, 1 out]
        n14 = local write "Stop"(w38) -> ()
      }
      frame "Update Sequence" {
        n15 = call-poly "Enqueue Message.vi"("error in (no error)"=w45, "Message Data"=w43, "Message"="Update Sequence", "Message Queue"=w46) -> ("error out"=w44:errorcluster)  [unwired: 6 in, 1 out]
      }
      frame "Pause Sequence" {
        n16 = call-poly "Enqueue Message.vi"("error in (no error)"=w50, "Message Data"=w48, "Message"="Pause", "Message Queue"=w51) -> ("error out"=w49:errorcluster)  [unwired: 6 in, 1 out]
      }
      frame "Resume Sequence" {
        n17 = call-poly "Enqueue Message.vi"("error in (no error)"=w55, "Message Data"=w53, "Message"="Resume", "Message Queue"=w56) -> ("error out"=w54:errorcluster)  [unwired: 6 in, 1 out]
      }
    }
  }
  n18 = while {
    tunnel: w10 -> [w79]
    tunnel: w9 -> [w78]
    shift-right: [w75] -> _
    shift-left: _ -> [w65]
    tunnel: [w73] -> w6
    shift-right: [w68] -> _
    shift-left: -1 -> [w70]
    shift-right: [w67] -> _
    shift-left: _ -> [w69]
    shift-right: [w63] -> _
    shift-left: -1 -> [w64]
    shift-right: [w62] -> _
    shift-left: _ -> [w61]
    tunnel: w3 -> [w60]
    shift-right: [w59] -> _
    shift-left: 0 -> [w58]
    stop <- w72 stop-if-true
    n19 = call "Dequeue Message.vi"("error in (no error)"=w78, "timeout in ms (-1)"=1, "Message Queue"=w79) -> ("error out"=w74:errorcluster, "Message Data"=w76:variant, "Message"=w77:string, "dup Message Queue"=w66:refnum<queue>)  [unwired: 5 in]
    n20 = case shown="\"Update Sequence\"" w77 {
      tunnel: w76 -> [_ w103 _ _ _ _ _]
      tunnel: [w87 w93 w109 w180 w189 w218 w545] -> w75
      tunnel: w74 -> [w86 w102 w110 w173 w182 w217 w544]
      tunnel: [w86 w95 w105 w173 w182 w205 w544] -> w73
      tunnel: [_ _ _ _ _ _ TRUE] -> w72
      tunnel: w65 -> [w87 _ w109 w180 w189 w199 w545]
      tunnel: w70 -> [w85 w100 _ w178 w187 w202 w543]
      tunnel: w69 -> [w84 w99 w111 w179 w188 w196 w542]
      tunnel: w64 -> [w82 w98 _ w176 w185 w209 w541]
      tunnel: [w85 w100 w107 w178 w187 w215 w543] -> w68
      tunnel: [w84 w99 w111 w179 w188 w212 w542] -> w67
      tunnel: w66 -> [_ _ _ _ _ w207 _]
      tunnel: [w82 w98 w107 w176 w185 w201 w541] -> w63
      tunnel: [w81 w97 FALSE w175 w184 w195 w540] -> w62
      tunnel: w61 -> [w81 w97 _ w175 w184 _ w540]
      tunnel: w60 -> [_ _ _ _ _ w193 _]
      tunnel: [w80 w94 w104 w172 w181 w192 w539] -> w59
      tunnel: w58 -> [w80 w94 w104 w172 w181 w191 w539]
      frame Default {
        n21 = Wait (ms)(milliseconds to wait=u32 10) -> ()  [unwired: 1 out]
      }
      frame "Update Sequence" {
        n22 = Variant To Data(error in=w102, type="Input", Variant=w103) -> (data=w93:T1, error out=w95:errorcluster)
        "Output" <- w93
        n23 = Unbundle By Name(w93) -> ("Main Config.Pump Module Configs"=w92:T38[])
        n24 = Index Array(array=w92, index=0) -> (element=w90:T38)
        n25 = Unbundle By Name(w90) -> ("Process Name"=→"Process Name":string, "Queue Name"=→"Queue Name":string)
        n26 = call "Write to Log File.vi"("error in"=w95, "text"="Sequencer: Update") -> ()  [unwired: 9 in, 1 out]
      }
      frame "Send Settings" {
        w107 = -1
        n27 = Unbundle By Name(w109) -> ("Main Config.Steps"=w113:T51)
        n28 = for {
          tunnel: w113 -> [w122] mode=indexing
          tunnel: [w117] -> w112 mode=indexing
          tunnel: w110 -> [w119]
          tunnel: w109 -> [w116]
          n29 = Unbundle By Name(w122) -> ("Module"=w121:string, "Control"=w114:u16, "Value"=w123:dbl)
          n30 = call "Find Queue (SubVI).vi"("Module"=w121, "Input"=w116) -> ("Found?"=w120:bool, "Queue out"=w115:refnum<queue>)  [unwired: 8 in]
          n31 = case shown="6" w114 {
            tunnel: [w157 w161 w165 w169] -> w118
            tunnel: w123 -> [w156 w160 w164 w168]
            frame 0, Default {
              n32 = Bundle By Name(cluster=T63 {"Auto?"=TRUE, "Manual Entry"=0.0, "Setpoint"=0.0}, "Auto?"=FALSE, "Manual Entry"=w156) -> (w157:T63)
            }
            frame 1 {
              n33 = Bundle By Name(cluster=T63 {"Auto?"=TRUE, "Manual Entry"=0.0, "Setpoint"=0.0}, "Auto?"=TRUE, "Setpoint"=w160) -> (w161:T63)
            }
            frame 5 {
              n34 = Bundle By Name(cluster=T63 {"Auto?"=TRUE, "Manual Entry"=0.0, "Setpoint"=0.0}, "Auto?"=TRUE, "Setpoint"=w164) -> (w165:T63)
            }
            frame 6 {
              n35 = Bundle By Name(cluster=T63 {"Auto?"=TRUE, "Manual Entry"=0.0, "Setpoint"=0.0}, "Auto?"=TRUE, "Setpoint"=w168) -> (w169:T63)
            }
          }
          n36 = case shown="False" w120 {
            tunnel: w119 -> [w124 w129]
            tunnel: w118 -> [_ w128]
            tunnel: [w124 w127] -> w117
            tunnel: w115 -> [_ w126]
            tunnel: w114 -> [_ w125]
            frame False {
            }
            frame True {
              n37 = case shown="Default" w125 {
                tunnel: w129 -> [w134 w135 w139 w149]
                tunnel: w128 -> [w133 _ w138 w148]
                tunnel: [w131 w135 w137 w147] -> w127
                tunnel: w126 -> [w130 _ w136 w146]
                frame Default {
                  n38 = call-poly "Enqueue Message.vi"("error in (no error)"=w134, "Message Data"=w133, "Message"="Sequence Update", "Message Queue"=w130) -> ("error out"=w131:errorcluster)  [unwired: 6 in, 1 out]
                }
                frame 3, 4, 7, 8 {
                }
                frame 5 {
                  n39 = disable-structure shown="Enabled" {
                    disable-tunnel: w139 -> [w144 w145]
                    disable-tunnel: w138 -> [w143 _]
                    disable-tunnel: [w141 w145] -> w137
                    disable-tunnel: w136 -> [w140 _]
                    frame Disabled {
                      n40 = call-poly "Enqueue Message.vi"("error in (no error)"=w144, "Message Data"=w143, "Message"="Sequence Update Speed", "Message Queue"=w140) -> ("error out"=w141:errorcluster)  [unwired: 6 in, 1 out]
                    }
                    frame Enabled {
                    }
                  }
                }
                frame 6 {
                  n41 = disable-structure shown="Enabled" {
                    disable-tunnel: w149 -> [w154 w155]
                    disable-tunnel: w148 -> [w153 _]
                    disable-tunnel: [w151 w155] -> w147
                    disable-tunnel: w146 -> [w150 _]
                    frame Disabled {
                      n42 = call-poly "Enqueue Message.vi"("error in (no error)"=w154, "Message Data"=w153, "Message"="Sequence Update Temperature", "Message Queue"=w150) -> ("error out"=w151:errorcluster)  [unwired: 6 in, 1 out]
                    }
                    frame Enabled {
                    }
                  }
                }
              }
            }
          }
          "Intruction Cluster" <- w122
        }
        n43 = Merge Errors(w112) -> (w105:errorcluster)
        n44 = call "Write to Log File.vi"("error in"=w105, "text"="Sequencer: Send Settings") -> ()  [unwired: 9 in, 1 out]
      }
      frame "Pause" {
        n45 = call "Write to Log File.vi"("error in"=w173, "text"="Sequencer: Pause") -> ()  [unwired: 9 in, 1 out]
        "Paused" <- TRUE ("Paused")
      }
      frame "Resume" {
        n46 = local write "Paused"(FALSE ("Paused")) -> ()
        n47 = call "Write to Log File.vi"("error in"=w182, "text"="Sequencer: Resume") -> ()  [unwired: 9 in, 1 out]
      }
      frame "Run Sequence" {
        n48 = Unbundle By Name(w199) -> ("Main Config.Steps"=w211:T51, "Main Config.Abort"=w190:bool)
        n49 = Less Than 0?(x=w202) -> (x < 0?=w203:bool)
        n50 = case shown="False" w203 {
          tunnel: [w537 0] -> w194
          tunnel: w202 -> [w537 _]
          frame False {
          }
          frame True {
          }
        }
        "Step" <- w194
        n51 = Array Size(array=w211) -> (size(s)=w210:i32)
        n52 = Equal?(x=w210, y=w209) -> (x = y?=w208:bool)
        n53 = Index Array(array=w211, index=w194) -> (element=w214:T52)
        n54 = Unbundle By Name(w214) -> ("Module"=w213:string, "Control"=w198:u16, "Value"=w197:dbl, "Wait (sec)"=w200:dbl)
        n55 = Not Equal?(x=w194, y=w209) -> (x != y?=w216:bool)
        n56 = case shown="True" w190 {
          tunnel: [w237 w533] -> w218
          tunnel: w217 -> [w236 w535]
          tunnel: w216 -> [w235 _]
          tunnel: [w234 w531] -> w215
          tunnel: w213 -> [w233 _]
          tunnel: [w232 w536] -> w212
          tunnel: w208 -> [w231 _]
          tunnel: [w230 w535] -> w206
          tunnel: [w229 w531] -> w201
          tunnel: w200 -> [w228 _]
          tunnel: w199 -> [w227 w533]
          tunnel: w198 -> [w226 _]
          tunnel: w197 -> [w225 _]
          tunnel: w196 -> [w224 w536]
          tunnel: [w223 TRUE] -> w195
          tunnel: w194 -> [w222 _]
          tunnel: w193 -> [w221 _]
          tunnel: [w220 0] -> w192
          tunnel: w191 -> [w219 _]
          frame False {
            n57 = case shown="True" w231 {
              tunnel: [w255 w529] -> w237
              tunnel: w236 -> [w246 w523]
              tunnel: w227 -> [w254 w529]
              tunnel: [w253 w523] -> w230
              tunnel: w235 -> [w252 _]
              tunnel: w222 -> [w251 w527]
              tunnel: [w250 w527] -> w234
              tunnel: w233 -> [w249 _]
              tunnel: w228 -> [w248 _]
              tunnel: [w247 w526] -> w232
              tunnel: [w245 w527] -> w229
              tunnel: w226 -> [w244 _]
              tunnel: w225 -> [w243 _]
              tunnel: w224 -> [w242 w526]
              tunnel: [FALSE w525] -> w223
              tunnel: w221 -> [w240 _]
              tunnel: [w239 0] -> w220
              tunnel: w219 -> [w238 _]
              frame False {
                # "Not Done"
                n58 = case shown="True" w252 {
                  tunnel: [w269 w428] -> w255
                  tunnel: w251 -> [w262 w418]
                  tunnel: w254 -> [w269 w428]
                  tunnel: [w259 w420] -> w253
                  tunnel: [w258 w417] -> w250
                  tunnel: w249 -> [w268 w419]
                  tunnel: w248 -> [w272 _]
                  tunnel: [w270 w422] -> w247
                  tunnel: w246 -> [w267 w425]
                  tunnel: [w262 w417] -> w245
                  tunnel: w244 -> [w263 w424]
                  tunnel: w243 -> [w266 w423]
                  tunnel: w242 -> [w270 _]
                  tunnel: w240 -> [w264 _]
                  tunnel: [w257 w415] -> w239
                  tunnel: w238 -> [w256 w416]
                  frame False {
                    # "Waiting for the next step"
                    n59 = local read "Paused"() -> (w271:bool)
                    n60 = case shown="False" w271 {
                      tunnel: [w284 w414] -> w258
                      tunnel: w262 -> [w283 w414]
                      tunnel: w272 -> [w282 _]
                      tunnel: w270 -> [w281 _]
                      tunnel: w263 -> [w280 _]
                      tunnel: w269 -> [w279 _]
                      tunnel: w268 -> [w275 _]
                      tunnel: w267 -> [w278 w413]
                      tunnel: [w277 w413] -> w260
                      tunnel: w266 -> [w276 _]
                      tunnel: [w274 w412] -> w257
                      tunnel: w256 -> [w273 w412]
                      frame False {
                        # "Paused?"
                        n61 = case shown="\"Default\", Default" w275 {
                          selector: w275 -> [_ _ w303]
                          tunnel: [w286 w296 w312] -> w284
                          tunnel: w283 -> [w287 w294 w311]
                          tunnel: w282 -> [_ _ w310]
                          tunnel: w281 -> [_ _ w309]
                          tunnel: w280 -> [_ _ w308]
                          tunnel: w279 -> [_ _ w307]
                          tunnel: w278 -> [w288 w295 w306]
                          tunnel: [w288 w295 w305] -> w277
                          tunnel: w276 -> [_ w292 w304]
                          tunnel: [w285 w291 w302] -> w274
                          tunnel: w273 -> [w285 w290 w302]
                          frame "Start Loop" {
                            n62 = Increment(x=w287) -> (x+1=w286:u32)
                            "Loop Variable" <- w287
                          }
                          frame "End Loop" {
                            n63 = Increment(x=w290) -> (x+1=w289:i32)
                            n64 = Less Or Equal?(x=w292, y=w289) -> (x <= y?=w293:bool)
                            n65 = case shown="False" w293 {
                              tunnel: [w298 w300] -> w296
                              tunnel: w294 -> [_ w301]
                              tunnel: [w297 w299] -> w291
                              tunnel: w289 -> [w297 w299]
                              frame False {
                                n66 = local read "Loop Variable"() -> (w298:u32)
                              }
                              frame True {
                                n67 = Increment(x=w301) -> (x+1=w300:u32)
                              }
                            }
                          }
                          frame "Default", Default {
                            n68 = case shown="0..2, 5, 6, Default" w308 {
                              tunnel: [w317 w332 w354 w376 w398] -> w312
                              tunnel: w311 -> [w316 w331 w353 w375 w397]
                              tunnel: w310 -> [w315 _ _ _ _]
                              tunnel: w309 -> [w314 _ _ _ _]
                              tunnel: w307 -> [_ w330 w352 w374 w396]
                              tunnel: w303 -> [_ w329 w351 w373 w395]
                              tunnel: w306 -> [w313 w326 w348 w370 w392]
                              tunnel: [w313 w325 w347 w369 w391] -> w305
                              tunnel: w304 -> [_ w324 w346 w368 w390]
                              frame 0..2, 5, 6, Default {
                                n69 = Get Date/Time In Seconds() -> (seconds since 1Jan1904=w320:timestamp)
                                n70 = Subtract(x=w320, y=w314) -> (x-y=w318:dbl)
                                n71 = Greater Or Equal?(x=w318, y=w315) -> (x >= y?=w319:bool)
                                n72 = case shown="True" w319 {
                                tunnel: w316 -> [w321 w323]
                                tunnel: [w321 w322] -> w317
                                frame False {
                                }
                                frame True {
                                # "Move to next step"
                                n73 = Increment(x=w323) -> (x+1=w322:u32)
                                }
                                }
                              }
                              frame 3 {
                                # "Wait Until Less Than"
                                n74 = call "Find Queue (SubVI).vi"("Module"=w329, "Input"=w330) -> ("Found?"=w328:bool, "Queue out"=w327:refnum<queue>)  [unwired: 8 in]
                                n75 = case shown="True" w328 {
                                tunnel: [w334 w342] -> w332
                                tunnel: w331 -> [w334 w341]
                                tunnel: w327 -> [_ w340]
                                tunnel: w326 -> [w333 w339]
                                tunnel: [w333 w338] -> w325
                                tunnel: w324 -> [_ w336]
                                frame False {
                                # "Error"
                                }
                                frame True {
                                n76 = call "Get Wait Until Data.vi"("error in (no error)"=w339, "Queue in"=w340) -> ("error out"=w338:errorcluster, "Data"=w337:dbl)  [unwired: 8 in]
                                n77 = Less Or Equal?(x=w337, y=w336) -> (x <= y?=w335:bool)
                                n78 = case shown="True" w335 {
                                tunnel: w341 -> [w343 w345]
                                tunnel: [w343 w344] -> w342
                                frame False {
                                }
                                frame True {
                                # "Move to next step"
                                n79 = Increment(x=w345) -> (x+1=w344:u32)
                                }
                                }
                                }
                                }
                              }
                              frame 4 {
                                # "Wait Until Greater Than"
                                n80 = call "Find Queue (SubVI).vi"("Module"=w351, "Input"=w352) -> ("Found?"=w350:bool, "Queue out"=w349:refnum<queue>)  [unwired: 8 in]
                                n81 = case shown="True" w350 {
                                tunnel: [w356 w364] -> w354
                                tunnel: w353 -> [w356 w363]
                                tunnel: w349 -> [_ w362]
                                tunnel: w348 -> [w355 w361]
                                tunnel: [w355 w360] -> w347
                                tunnel: w346 -> [_ w358]
                                frame False {
                                # "Error"
                                }
                                frame True {
                                n82 = call "Get Wait Until Data.vi"("error in (no error)"=w361, "Queue in"=w362) -> ("error out"=w360:errorcluster, "Data"=w359:dbl)  [unwired: 8 in]
                                n83 = Greater Or Equal?(x=w359, y=w358) -> (x >= y?=w357:bool)
                                n84 = case shown="True" w357 {
                                tunnel: w363 -> [w365 w367]
                                tunnel: [w365 w366] -> w364
                                frame False {
                                }
                                frame True {
                                # "Move to next step"
                                n85 = Increment(x=w367) -> (x+1=w366:u32)
                                }
                                }
                                }
                                }
                              }
                              frame 7 {
                                # "Wait Until TCU is Less Than"
                                n86 = call "Find Queue (SubVI).vi"("Module"=w373, "Input"=w374) -> ("Found?"=w372:bool, "Queue out"=w371:refnum<queue>)  [unwired: 8 in]
                                n87 = case shown="True" w372 {
                                tunnel: [w378 w386] -> w376
                                tunnel: w375 -> [w378 w385]
                                tunnel: w371 -> [_ w384]
                                tunnel: w370 -> [w377 w383]
                                tunnel: [w377 w382] -> w369
                                tunnel: w368 -> [_ w380]
                                frame False {
                                # "Error"
                                }
                                frame True {
                                n88 = call "Get Wait Until Data.vi"("error in (no error)"=w383, "Queue in"=w384) -> ("error out"=w382:errorcluster, "Data"=w381:dbl)  [unwired: 8 in]
                                n89 = Less Or Equal?(x=w381, y=w380) -> (x <= y?=w379:bool)
                                n90 = case shown="True" w379 {
                                tunnel: w385 -> [w387 w389]
                                tunnel: [w387 w388] -> w386
                                frame False {
                                }
                                frame True {
                                # "Move to next step"
                                n91 = Increment(x=w389) -> (x+1=w388:u32)
                                }
                                }
                                }
                                }
                              }
                              frame 8 {
                                # "Wait Until TCU is Greater Than"
                                n92 = call "Find Queue (SubVI).vi"("Module"=w395, "Input"=w396) -> ("Found?"=w394:bool, "Queue out"=w393:refnum<queue>)  [unwired: 8 in]
                                n93 = case shown="True" w394 {
                                tunnel: [w400 w408] -> w398
                                tunnel: w397 -> [w400 w407]
                                tunnel: w393 -> [_ w406]
                                tunnel: w392 -> [w399 w405]
                                tunnel: [w399 w404] -> w391
                                tunnel: w390 -> [_ w402]
                                frame False {
                                # "Error"
                                }
                                frame True {
                                n94 = call "Get Wait Until Data.vi"("error in (no error)"=w405, "Queue in"=w406) -> ("error out"=w404:errorcluster, "Data"=w403:dbl)  [unwired: 8 in]
                                n95 = Greater Or Equal?(x=w403, y=w402) -> (x >= y?=w401:bool)
                                n96 = case shown="True" w401 {
                                tunnel: w407 -> [w409 w411]
                                tunnel: [w409 w410] -> w408
                                frame False {
                                }
                                frame True {
                                # "Move to next step"
                                n97 = Increment(x=w411) -> (x+1=w410:u32)
                                }
                                }
                                }
                                }
                              }
                            }
                          }
                        }
                      }
                      frame True {
                        # "Paused?"
                      }
                    }
                    n98 = call-poly "Enqueue Message.vi"("Message Data"=w258, "Message"="Update Step", "Message Queue"=w264) -> ("error out"=w261:errorcluster)  [unwired: 7 in, 1 out]
                    n99 = Merge Errors(w260, w261) -> (w259:errorcluster)
                  }
                  frame True {
                    # "Moved to the next step"
                    n100 = call "Find Queue (SubVI).vi"("Module"=w419, "Input"=w428) -> ("Found?"=w427:bool, "Queue out"=w426:refnum<queue>)  [unwired: 8 in]
                    n101 = case shown="False" w427 {
                      tunnel: w426 -> [_ w460]
                      tunnel: w425 -> [w435 w459]
                      tunnel: [w434 w458] -> w420
                      tunnel: w424 -> [_ w462]
                      tunnel: w423 -> [w430 w461]
                      tunnel: w419 -> [w436 _]
                      tunnel: w418 -> [w433 w457]
                      tunnel: [w432 w457] -> w417
                      tunnel: w416 -> [w431 w456]
                      tunnel: [w429 w456] -> w415
                      frame False {
                        # "Queue not found. ERROR"
                        n102 = case shown="\"End Loop\"" w436 {
                          tunnel: [w439 w446 w455] -> w434
                          tunnel: w435 -> [w439 w446 w455]
                          tunnel: w433 -> [w438 w442 w454]
                          tunnel: [w438 w447 w454] -> w432
                          tunnel: w431 -> [w437 w444 w453]
                          tunnel: w430 -> [_ w445 _]
                          tunnel: [w437 w441 w453] -> w429
                          frame "Start Loop" {
                            n103 = local write "Loop Variable"(w438) -> ()
                          }
                          frame "End Loop" {
                            n104 = Increment(x=w444) -> (x+1=w440:i32)
                            n105 = Less Or Equal?(x=w445, y=w440) -> (x <= y?=w443:bool)
                            n106 = case shown="True" w443 {
                              tunnel: [w449 w451] -> w447
                              tunnel: w442 -> [_ w452]
                              tunnel: [w448 0] -> w441
                              tunnel: w440 -> [w448 _]
                              frame False {
                                n107 = local read "Loop Variable"() -> (w449:u32)
                              }
                              frame True {
                                n108 = Increment(x=w452) -> (x+1=w451:u32)
                              }
                            }
                          }
                          frame "Default", Default {
                            # "Error"
                          }
                        }
                      }
                      frame True {
                        # "Queue Found"
                        n109 = case shown="0" w462 {
                          tunnel: w461 -> [w471 w482 w493 w504 w514 _ _]
                          tunnel: w460 -> [w469 w479 w490 w501 w512 _ w520]
                          tunnel: w459 -> [w467 w478 w489 w500 w513 w517 w519]
                          tunnel: [w463 w474 w485 w496 w507 w517 w518] -> w458
                          frame 0 {
                            # "Manual"
                            n110 = Bundle By Name(cluster=T63 {"Auto?"=TRUE, "Manual Entry"=0.0, "Setpoint"=0.0}, "Auto?"=FALSE, "Manual Entry"=w471) -> (w468:T63)
                            n111 = call-poly "Enqueue Message.vi"("error in (no error)"=w467, "Message Data"=w468, "Message"="Sequence Update", "Message Queue"=w469) -> ("error out"=w465:errorcluster, "dup Message Queue"=w466:refnum<queue>)  [unwired: 6 in]
                            n112 = call-poly "Enqueue Message.vi"("error in (no error)"=w465, "Message"="Sequence Start", "Message Queue"=w466) -> ("error out"=w463:errorcluster)  [unwired: 7 in, 1 out]
                          }
                          frame 1 {
                            # "Auto"
                            n113 = Bundle By Name(cluster=T63 {"Auto?"=TRUE, "Manual Entry"=0.0, "Setpoint"=0.0}, "Auto?"=TRUE, "Setpoint"=w482) -> (w480:T63)
                            n114 = call-poly "Enqueue Message.vi"("error in (no error)"=w478, "Message Data"=w480, "Message"="Sequence Update", "Message Queue"=w479) -> ("error out"=w476:errorcluster, "dup Message Queue"=w475:refnum<queue>)  [unwired: 6 in]
                            n115 = call-poly "Enqueue Message.vi"("error in (no error)"=w476, "Message"="Sequence Start", "Message Queue"=w475) -> ("error out"=w474:errorcluster)  [unwired: 7 in, 1 out]
                          }
                          frame 5 {
                            # "Update TCU Speed"
                            n116 = Bundle By Name(cluster=T63 {"Auto?"=TRUE, "Manual Entry"=0.0, "Setpoint"=0.0}, "Auto?"=TRUE, "Setpoint"=w493) -> (w491:T63)
                            n117 = call-poly "Enqueue Message.vi"("error in (no error)"=w489, "Message Data"=w491, "Message"="Sequence Update Speed", "Message Queue"=w490) -> ("error out"=w487:errorcluster, "dup Message Queue"=w486:refnum<queue>)  [unwired: 6 in]
                            n118 = call-poly "Enqueue Message.vi"("error in (no error)"=w487, "Message"="Sequence Start", "Message Queue"=w486) -> ("error out"=w485:errorcluster)  [unwired: 7 in, 1 out]
                          }
                          frame 6 {
                            # "Update TCU Tempurature"
                            n119 = Bundle By Name(cluster=T63 {"Auto?"=TRUE, "Manual Entry"=0.0, "Setpoint"=0.0}, "Auto?"=TRUE, "Setpoint"=w504) -> (w502:T63)
                            n120 = call-poly "Enqueue Message.vi"("error in (no error)"=w500, "Message Data"=w502, "Message"="Sequence Update Temperature", "Message Queue"=w501) -> ("error out"=w498:errorcluster, "dup Message Queue"=w497:refnum<queue>)  [unwired: 6 in]
                            n121 = call-poly "Enqueue Message.vi"("error in (no error)"=w498, "Message"="Sequence Start", "Message Queue"=w497) -> ("error out"=w496:errorcluster)  [unwired: 7 in, 1 out]
                          }
                          frame 2 {
                            # "DIO"
                            n122 = Bundle By Name(cluster=T63 {"Auto?"=TRUE, "Manual Entry"=0.0, "Setpoint"=0.0}, "Setpoint"=w514) -> (w511:T63)
                            n123 = call-poly "Enqueue Message.vi"("error in (no error)"=w513, "Message Data"=w511, "Message"="Sequence Update", "Message Queue"=w512) -> ("error out"=w508:errorcluster, "dup Message Queue"=w509:refnum<queue>)  [unwired: 6 in]
                            n124 = call-poly "Enqueue Message.vi"("error in (no error)"=w508, "Message"="Sequence Start", "Message Queue"=w509) -> ("error out"=w507:errorcluster)  [unwired: 7 in, 1 out]
                          }
                          frame 3, 4 {
                            # "Wait until"
                          }
                          frame Default {
                            n125 = call-poly "Enqueue Message.vi"("error in (no error)"=w519, "Message"="Sequence Start", "Message Queue"=w520) -> ("error out"=w518:errorcluster)  [unwired: 7 in, 1 out]
                          }
                        }
                      }
                    }
                    n126 = Get Date/Time In Seconds() -> (seconds since 1Jan1904=w422:timestamp)
                    n127 = call "Write to Log File.vi"("error in"=w420, "text"="Sequencer: Next Step") -> ()  [unwired: 9 in, 1 out]
                  }
                }
              }
              frame True {
                w525 = TRUE
                # "Done"
                n128 = Wait (ms)(milliseconds to wait=u32 100) -> ()  [unwired: 1 out]
                n129 = call "Write to Log File.vi"("error in"=w523, "text"="Sequencer: Done") -> ()  [unwired: 9 in, 1 out]
                "Done" <- w525
              }
            }
          }
          frame True {
            n130 = Unbundle By Name(w533) -> ("Main Config.Steps"=w532:T51)
            n131 = Array Size(array=w532) -> (size(s)=w531:i32)
          }
        }
        n132 = call-poly "Enqueue Message.vi"("error in (no error)"=w206, "Message"="Run Sequence", "Message Queue"=w207) -> ("error out"=w205:errorcluster)  [unwired: 7 in, 1 out]
      }
      frame "Exit" {
      }
    }
  }
  n133 = Merge Errors(w8, w6) -> (→"error out":errorcluster)
